vi "gyro rate safety.vi"(6 "Encoder Failure":bool, 8 "Cutoff Rate":dbl=0.2, 9 "Input":dbl, 10 "Gyro Angular Rate":dbl, 11 "Encoder Rate":dbl) -> (0 "No Gyro Rate Read":bool, 1 "Gyro Failure":bool, 2 "Output":dbl, 3 "Gyro Angular Rate Out":dbl)   [LabVIEW 2014]
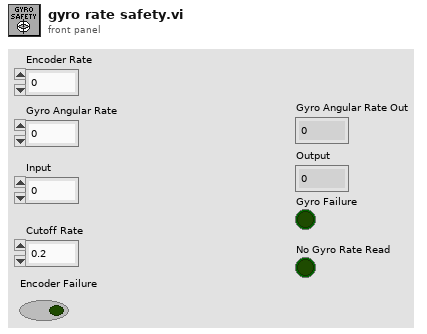
[diagram p1: front panel]
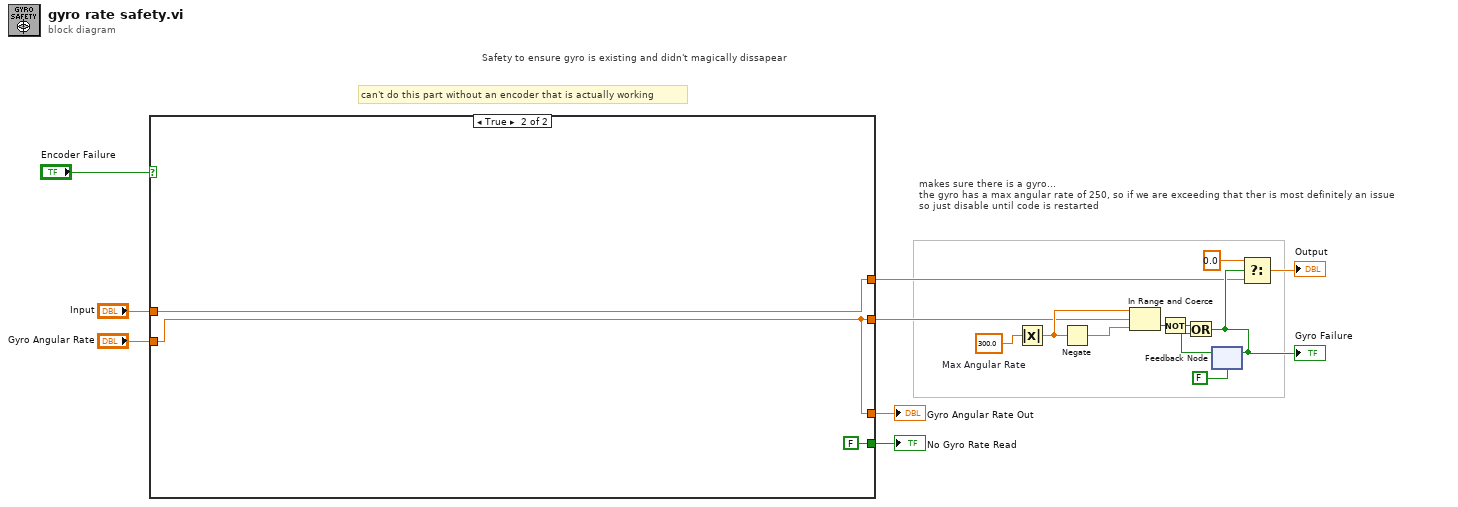
[diagram p0: block diagram]
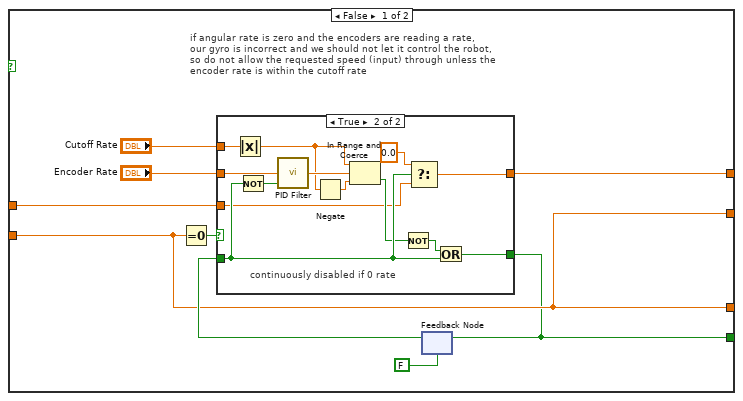
[diagram p2: hidden frame]
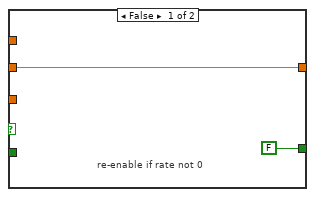
[diagram p3: hidden frame]
diagram:
  w7 = 300.0  # Max Angular Rate
  # "can't do this part without an encoder that is actually working"
  # "makes sure there is a gyro...\nthe gyro has a max angular rate of 250, so if we are exceeding that ther is most definitely an issue\nso just disable until code is restarted"
  # "Safety to ensure gyro is existing and didn't magically dissapear"
  n1 = case shown="True" "Encoder Failure" {
    tunnel: [w23 w44] -> w15
    tunnel: [w19 w42] -> w6
    tunnel: "Input" -> [w20 w44]
    tunnel: "Gyro Angular Rate" -> [w19 w42]
    tunnel: [w19 w42] -> w2
    tunnel: [w18 FALSE] -> w1
    frame False {
      # "if angular rate is zero and the encoders are reading a rate,\nour gyro is incorrect and we should not let it control the robot,\nso do not allow the requested speed (input) through unless the\nencoder rate is within the cutoff rate"
      n2 = Equal To 0?(x=w19) -> (x = 0?=w26:bool)
      n3 = feedback #1(FALSE ("x > y?")) -> (w24:bool)
      n4 = case shown="True" w26 {
        tunnel: "Encoder Rate" -> [w28 w31]
        tunnel: [w28 w40] -> w23
        tunnel: [FALSE w38] -> w18
        tunnel: w24 -> [_ w37]
        tunnel: "Cutoff Rate" -> [_ w35]
        tunnel: w20 -> [_ w29]
        frame False {
          # "re-enable if rate not 0"
        }
        frame True {
          # "continuously disabled if 0 rate"
          n5 = Absolute Value(x=w35) -> (abs(x)=w30:dbl)
          n6 = Not(x=w37) -> (.not. x?=w34:bool)
          n7 = call "PID Filter.vi"("reinitialize? (F)"=w34, "input"=w31) -> ("output"=w33:dbl)  [unwired: 3 in]
          n8 = Negate(x=w30) -> (-x=w36:dbl)
          n9 = In Range and Coerce(upper limit=w30, x=w33, lower limit=w36) -> (In Range?=w32:bool)  [unwired: 1 out]
          n10 = Not(x=w32) -> (.not. x?=w39:bool)
          n11 = Select(t=0.0, s=w37, f=w29) -> (s? t:f=w40:dbl)
          n12 = Or(x=w39, y=w37) -> (x .or. y?=w38:bool)
        }
      }
      n13 = feedback-in #1(w18) -> ()
    }
    frame True {
    }
  }
  "Gyro Angular Rate Out" <- w2
  "No Gyro Rate Read" <- w1
  n14 = Absolute Value(x=w7) -> (abs(x)=w8:dbl)
  n15 = Negate(x=w8) -> (-x=w9:dbl)
  n16 = In Range and Coerce(upper limit=w8, x=w6, lower limit=w9) -> (In Range?=w11:bool)  [unwired: 1 out]
  n17 = Not(x=w11) -> (.not. x?=w10:bool)
  n18 = feedback #2(FALSE ("x > y?")) -> (w12:bool)
  n19 = Or(x=w10, y=w12) -> (x .or. y?=w17:bool)
  "Gyro Failure" <- w17
  n20 = feedback-in #2(w17) -> ()
  n21 = Select(t=0.0, s=w17, f=w15) -> (s? t:f=→"Output":dbl)
